vi "startCamera.vi"(8 "error in (no error)":errorcluster, 10 "camera":string, 11 "AtomChipHWC in":refnum<class "AtomChipHWC.lvclass">) -> (0 "error out":errorcluster, 3 "AtomChipHWC out":refnum<class "AtomChipHWC.lvclass">)   [LabVIEW 2009, in "Hardware.lvlib" / "HWControllers.lvlib" / "AtomChipHWC.lvclass"]
uses:
  AtomChipHWC.lvclass
  AtomChipHWC.lvclass/AtomChipHWC.ctl
  Network Controllers/NetworkCamera/NetworkCamera.lvclass
  IntegrationManagement/CameraManager.lvclass
  Network Controllers/CameraNetworkController/CameraNetworkController.lvclass
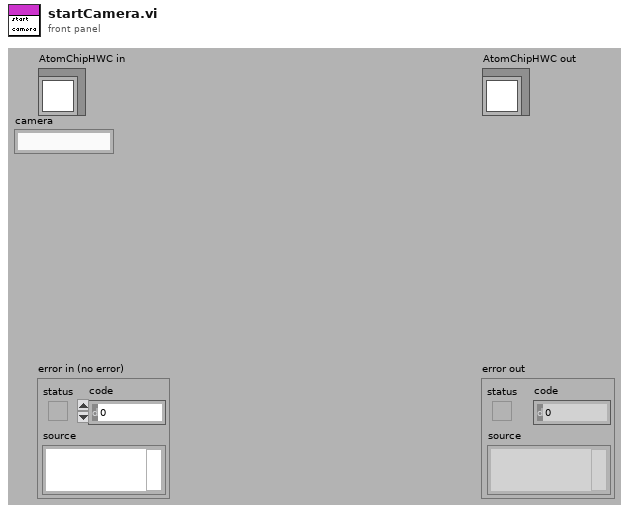
[diagram p1: front panel]
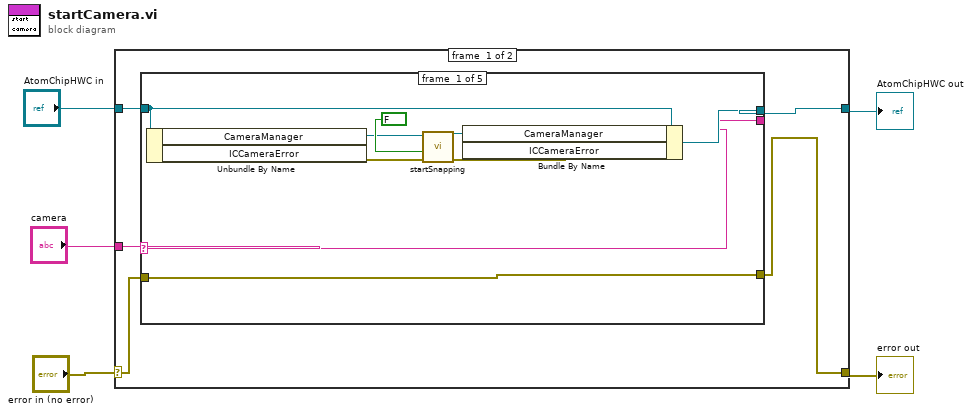
[diagram p0: block diagram]
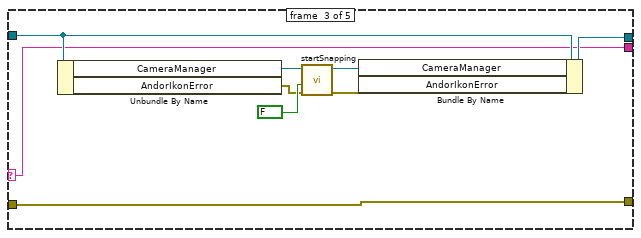
[diagram p3: hidden frame]
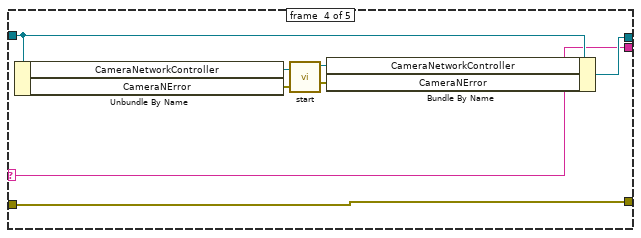
[diagram p4: hidden frame]
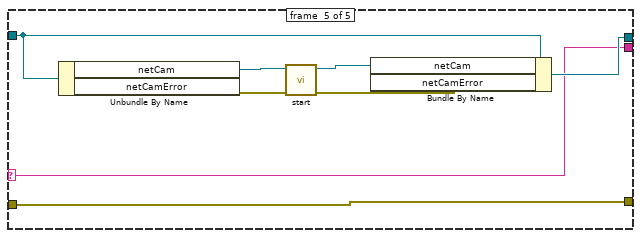
[diagram p5: hidden frame]
diagram:
  n1 = case shown="No Error" "error in (no error)" {
    selector: "error in (no error)" -> [w8 w48]
    tunnel: [w6 w48] -> w4
    tunnel: [w7 w47] -> w2
    tunnel: "AtomChipHWC in" -> [w9 w47]
    tunnel: "camera" -> [w10 _]
    frame #0 {
      n2 = case shown="\"Pixelfly\", \"ProEM_WinX32\"" w10 {
        selector: w10 -> [w14 _ w25 w34 w44]
        tunnel: w9 -> [w15 w21 w29 w37 w46]
        tunnel: w8 -> [w11 w20 w22 w31 w43]
        tunnel: [w11 w20 w22 w31 w43] -> w6
        tunnel: [w16 w21 w26 w35 w45] -> w7
        tunnel: [w14 _ w25 w34 w44] -> _
        frame #0 {
          n3 = Unbundle By Name(w15) -> ("CameraManager"=w18:refnum<class "CameraManager.lvclass">, "ICCameraError"=w13:errorcluster)
          n4 = call "startSnapping.vi"("error in (no error)"=w13, "releaseWhenReady"=FALSE, "CameraManager in"=w18) -> ("error out"=w12:errorcluster, "CameraManager out"=w17:refnum<class "CameraManager.lvclass">)  [unwired: 7 in]
          n5 = Bundle By Name(cluster=w15, "CameraManager"=w17, "ICCameraError"=w12) -> (w16:refnum<class "AtomChipHWC.lvclass">)
        }
        frame #1 {
        }
        frame #2 {
          n6 = Unbundle By Name(w29) -> ("CameraManager"=w30:refnum<class "CameraManager.lvclass">, "AndorIkonError"=w24:errorcluster)
          n7 = call "startSnapping.vi"("error in (no error)"=w24, "releaseWhenReady"=FALSE, "CameraManager in"=w30) -> ("error out"=w23:errorcluster, "CameraManager out"=w28:refnum<class "CameraManager.lvclass">)  [unwired: 7 in]
          n8 = Bundle By Name(cluster=w29, "CameraManager"=w28, "AndorIkonError"=w23) -> (w26:refnum<class "AtomChipHWC.lvclass">)
        }
        frame #3 {
          n9 = Unbundle By Name(w37) -> ("CameraNetworkController"=w38:refnum<class "CameraNetworkController.lvclass">, "CameraNError"=w33:errorcluster)
          n10 = call "start.vi"("error in (no error)"=w33, "CameraNetworkController in"=w38) -> ("error out"=w32:errorcluster, "CameraNetworkController out"=w36:refnum<class "CameraNetworkController.lvclass">)  [unwired: 8 in]
          n11 = Bundle By Name(cluster=w37, "CameraNetworkController"=w36, "CameraNError"=w32) -> (w35:refnum<class "AtomChipHWC.lvclass">)
        }
        frame #4 {
          n12 = Unbundle By Name(w46) -> ("netCam"=w42:refnum<class "NetworkCamera.lvclass">, "netCamError"=w40:errorcluster)
          n13 = call-dynamic "start.vi"("error in (no error)"=w40, "NetworkCamera in"=w42) -> ("error out"=w39:errorcluster, "NetworkCamera out"=w41:refnum<class "NetworkCamera.lvclass">)  [unwired: 8 in]
          n14 = Bundle By Name(cluster=w46, "netCam"=w41, "netCamError"=w39) -> (w45:refnum<class "AtomChipHWC.lvclass">)
        }
      }
    }
    frame #1 {
    }
  }
  "error out" <- w4
  "AtomChipHWC out" <- w2
